vi "GT Load Config.vi"(8 "error in (no error)":errorcluster caption="错误输入（无错误）", 10 "pFile":string, 11 "cardNum":i16) -> (0 "error out":errorcluster caption="错误输出", 2 "pFile out":string, 3 "function return":i16)   [LabVIEW 2014, in "gts.lvlib"]
doc: "GT_API GT_LoadConfig(short cardNum,char *pFile);"
uses:
  gts.lvlib
  gts.dll
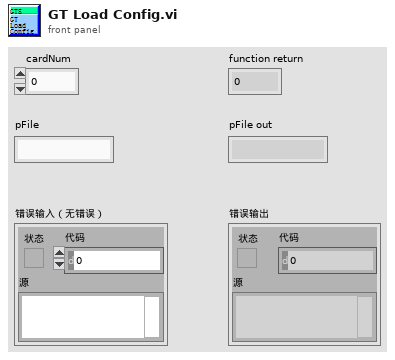
[diagram p1: front panel]
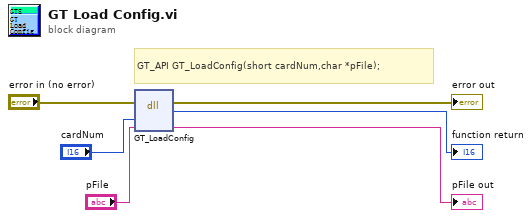
[diagram p0: block diagram]
diagram:
  # "GT_API GT_LoadConfig(short cardNum,char *pFile);"
  n1 = dll-call lib="PTH2>abs F.多卡库-控制卡基本运动例程(labview)gts.*" fn="GT_LoadConfig"(error in="error in (no error)", "cardNum"="cardNum", "pFile"="pFile") -> (error out=→"error out":errorcluster, →"function return":i16, "pFile"=→"pFile out":string)  [unwired: 3 in, 1 out]
